vi "NI 5772 (AC) - TIS Mode Enabled (FPGA).vi"() -> ()   [LabVIEW 2018]
doc: "Example Description:\nThis example demonstrates how to enable Time Interleaved Sampling with the NI 5772 adapter module to achieve a sampling rate of 1.6GS/s. This example continuously acquires records of analog input data from the NI 5772 adapter module. It allows you to select an AI channel, trigger type, and record size. This VI must be compiled before it is run. \n\nRunning the VI:\nThis VI must be run from the NI 5772 - Getting Started (Host).vi. Refer to the host VI documentation for steps regarding running and configuring the FPGA VI. \n\nExecution Steps:\nRefer to the Block Diagram of this VI for execution comments."
uses:
  Controls/AI Trigger Type.ctl
  Controls/Aquire State.ctl
  <vilib>/Platform/TimedLoop/XDataNode/timing_clust.ctl
  <vilib>/Platform/TimedLoop/XDataNode/nitl_modes.ctl
  <vilib>/Platform/TimedLoop/XDataNode/wakeup.ctl
  E:/Norway Project/All Hardware/New Microscope/LabVIEW/HardwareRevamp/AcustoXv2/Controls/DigitizerState.ctl
  <instrlib>/_niInstr/Data Trigger/v1/Shared/Public/Edge Configuration Bool.ctl
  <instrlib>/_niInstr/Data Trigger/v1/Shared/Public/Edge Configuration Trigger Slope.ctl
  <vilib>/rvi/Emulation/niFpgaGetClockAttributes.vi
  <vilib>/rvi/Emulation/niFpgaSctlEmulationGetInTimedLoop.vi
  <vilib>/rvi/Emulation/niFpgaEmulationReportErrorSimple.vi
  <vilib>/rvi/eio/common/nirviEmuTemplateMethod_errors.vi
  <vilib>/rvi/Emulation/niFpgaCriticalErrorInLSC.vi
  <vilib>/rvi/Emulation/niFpgaProcessEmulError.vi
  <instrlib>/_niInstr/Data Trigger/v1/FPGA/Private/Trigger/Edge Boolx1spc.vi
  <vilib>/rvi/Emulation/niFpgaEmulationIsFPGAContextNoSignature.vi
  <vilib>/rvi/errors/niFpgaSetErrorForExecOnDevCompSimple.vi
  <vilib>/rvi/eio/common/nirviEmuReportErrorAndStop.vi
  <vilib>/rvi/DataTransferAndStorage/Container/Common/niFpgaContainerGetUniqueNameForEmu.vi
  <vilib>/rvi/FIFO/Fifo_Resource/nirvififoEmulationSetSize.vi
  <vilib>/rvi/FIFO/Fifo_Resource/nirviFifoEmulationQueueMgr.vi
  <instcachedir>/0/nirviFifoEmulationQueueMgr_E5CAEC123FF24DC58D834DCA3CDAA9B5.lvgen/nirviFifoEmulationQueueMgr_E5CAEC123FF24DC58D834DCA3CDAA9B5_003.vi
  <vilib>/rvi/FIFO/Fifo_Resource/nirvififoEmulationDetermineInputValidOut.vi
  <vilib>/rvi/FIFO/Fifo_Resource/nirvififoEmulationCreateLock.vi
  <vilib>/rvi/FIFO/Fifo_Resource/nirvififoEmulationObtainLock.vi
  <vilib>/rvi/FIFO/Fifo_Resource/nirvififoEmulationReleaseLock.vi
  <vilib>/rvi/occurrence/nirviWaitOnOccurrenceBase.vi
  <vilib>/rvi/errors/nirviReportUnexpectedCaseInternalError.vi
  <vilib>/rvi/errors/nirviReportUnexpectedCaseInternalError (U32).vi
  <vilib>/Utility/error.llb/Clear Errors.vi
  <vilib>/rvi/interface/RandomDataEmulation/niFpgaRandomDataHandleErrors.vi
  <vilib>/eio/EIONode/EIONode.xnode
  <vilib>/Platform/TimedLoop/XDataNode/XDataNode.xnode
  <vilib>/rvi/DataTransferAndStorage/Container/XNode/niFpgaContainer.xnode
  <vilib>/rvi/FIFO/Fifo_Resource/nirvififoEmulationWrite.vi
  <vilib>/rvi/FIFO/Fifo_Resource/nirvififoEmulationRead.vi
  <vilib>/rvi/interface/RandomDataEmulation/nirviRandomDataFpgaReadWriteTemplate.vi
  <vilib>/Platform/TimedLoop/XDataNode/XDNodeRunTimeDep.lvlib
  <instrlib>/_niInstr/Data Trigger/v1/FPGA/niInstr Data Trigger v1 FPGA.lvlib
  <instrlib>/_niInstr/Data Trigger/v1/Shared/niInstr Data Trigger v1 Shared.lvlib
panel:
  in  "vi/nGenTrig":bool
  out "Pixel and Wave":T1
  out "Completed?":bool
  in  "Scan Mode":enum16{"Raster Scan", "Serpentine Scan"}(ring)
  in  "Line Count":u16
  in  "Pixel Count":u16
  in  "TrigIn Simulate":bool
  in  "Filteration":bool
  out "DMA FIFO Overflow?":bool caption="FIFO Overflow?"
  in  "AvgCount":u16=1
  in  "Delay after Trig [us]":sgl
  out "Delay after Trig [cycles]":u16
  out "TS FIFO In Overflow?":bool caption="FIFO Overflow?"
  in  "Samples Per Trigger":u16=512 min=1 step=1
  in  "Arm Trigger":bool
  in  "User Command Commit":bool
  in  "User Command":u8
  out "User Command Idle":bool
  out "User Command Status":u8
  in  "User Data 0":u16
  in  "User Data 1":u8
  out "PLL Locked":bool
  out "User Error":bool
  out "Configured?":bool
  in  "Trigger Level":i16
  in  "Trigger Type":T2
  # "Resource Configuration"
  # "Analog Input"
  # "Clock Configuration"
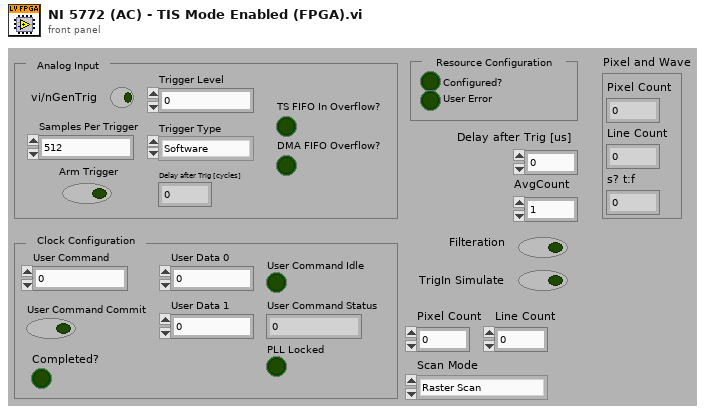
[diagram p1: front panel]
types:
  T1 = cluster{"Pixel Count":i32, "Line Count":u16, "s? t:f":u64}
  T2 = typedef "AI Trigger Type.ctl" = enum8{"Software", "Data Edge"}
  T3 = typedef "DigitizerState.ctl" = enum16{"GetData", "Filter", "AverageCountCheck", "SendtoHost", "CompleteScan"}
  T4 = typedef "Aquire State.ctl" = enum8{"Idle", "Wait for Trigger", "Hold Aquire", "Acquire"}
  T5 = typedef "XDNodeRunTimeDep.lvlib/timing_clust.ctl" = cluster{"Expected End [f-1]":u64, "Actual End [f-1]":u64, "Finished Late? [f-1]":bool, "Expected End [i-1]":u64, "Actual End [i-1]":u64, "Finished Late? [i-1]":bool, "Expected Start [i]":u64, "Actual Start [i]":u64, "Expected Start [f]":u64, "Actual Start [f]":u64, "Source Name":string, "Structure Name":string, "Period":i64, "Deadline":i64, "Offset":i64, "Start":i64, "Priority":i32, "Timeout":i32, "Mode":T6, "Wakeup Reason":T7, "Error":errorcluster, "Source Type":string, "Secondary Source Type":string, "Global End Time":u64, "Global Start Time":u64, "Frame Duration":u64, "Iteration Duration":u64, "Assigned CPU":i32, "I/O Scan Engine Mode":u32}
  T6 = typedef "XDNodeRunTimeDep.lvlib/nitl_modes.ctl" = enum32{"No Change", "Process missed periods, maintain original phase", "Discard missed periods, maintain original phase", "Process missed periods, ignore original phase", "Discard missed periods, ignore original phase"}
  T7 = typedef "XDNodeRunTimeDep.lvlib/wakeup.ctl" = enum32{"Normal", "Aborted", "Asynchronous wakeup", "Timing source error", "Timed loop error", "Timeout"}
  T8 = typedef "niInstr Data Trigger v1 Shared.lvlib/Edge Configuration Bool.ctl" = cluster{"trigger slope":T9}
  T9 = typedef "niInstr Data Trigger v1 Shared.lvlib/Edge Configuration Trigger Slope.ctl" = enum8{"Positive", "Negative"}
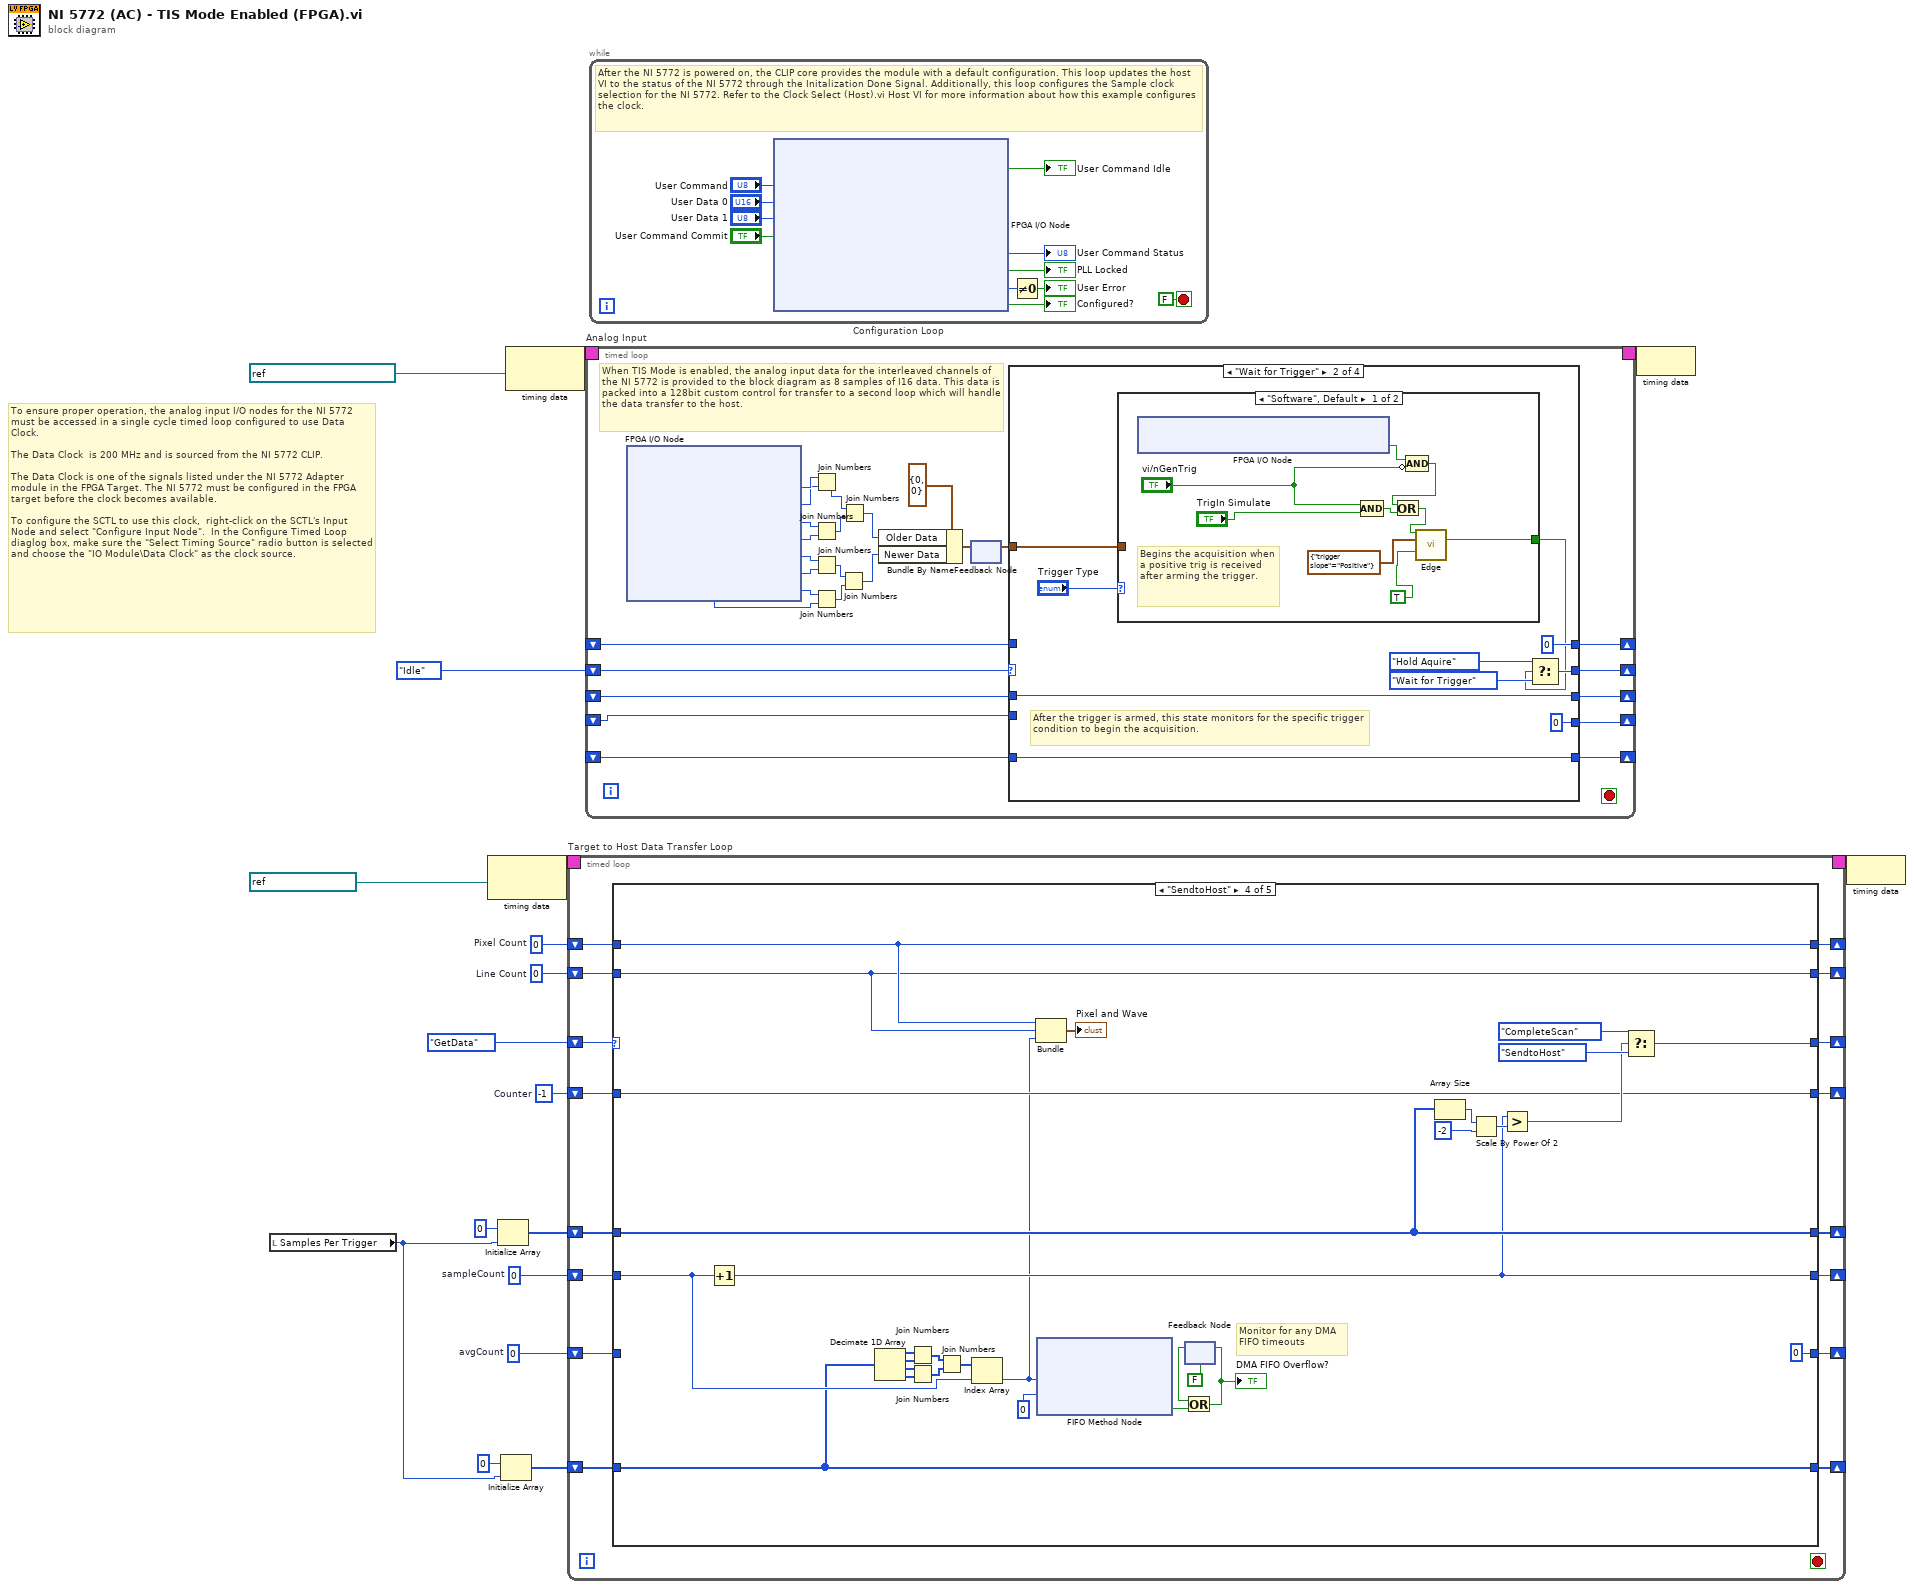
[diagram p0: block diagram]
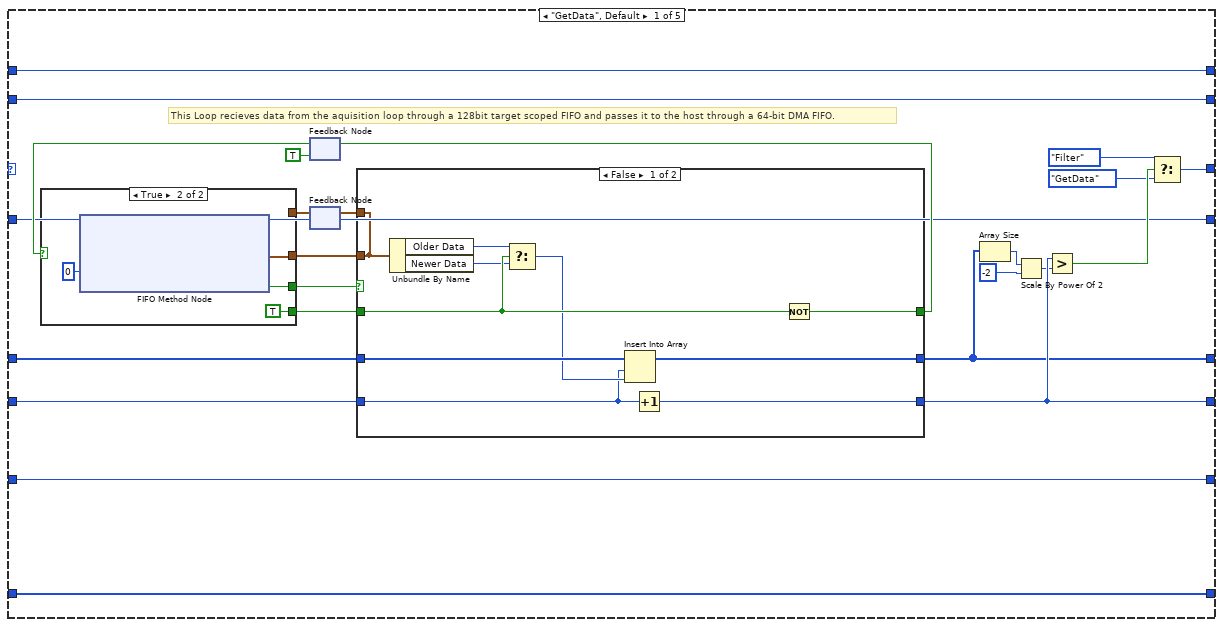
[diagram p2: hidden frame]
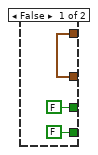
[diagram p3: hidden frame]
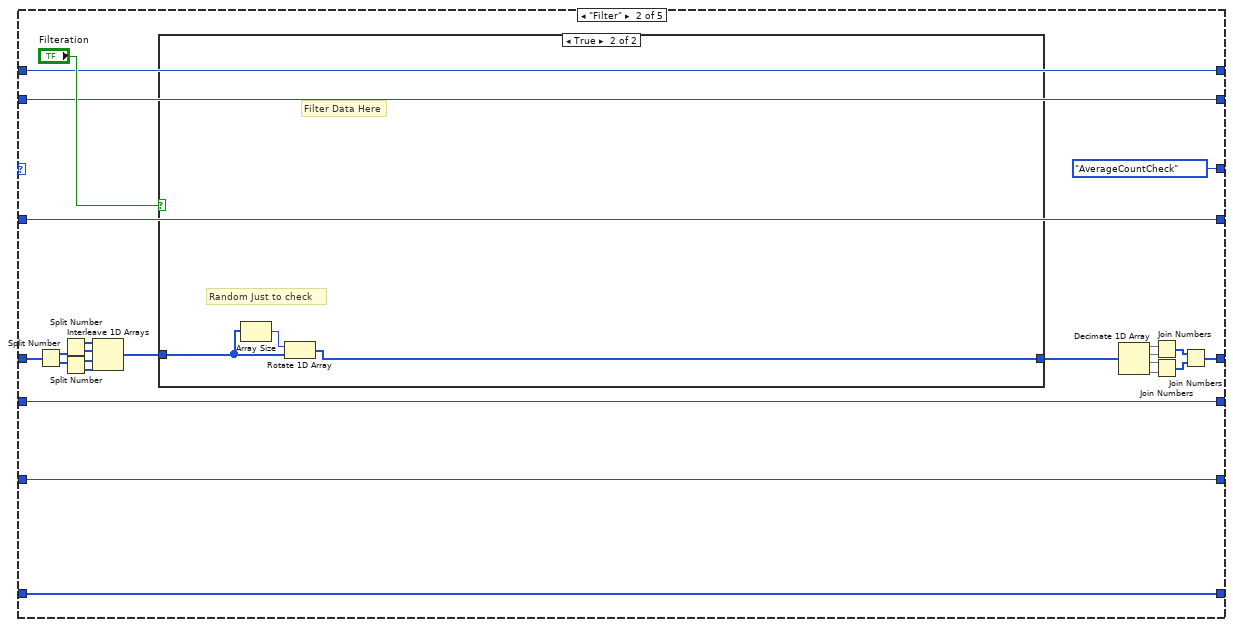
[diagram p5: hidden frame]
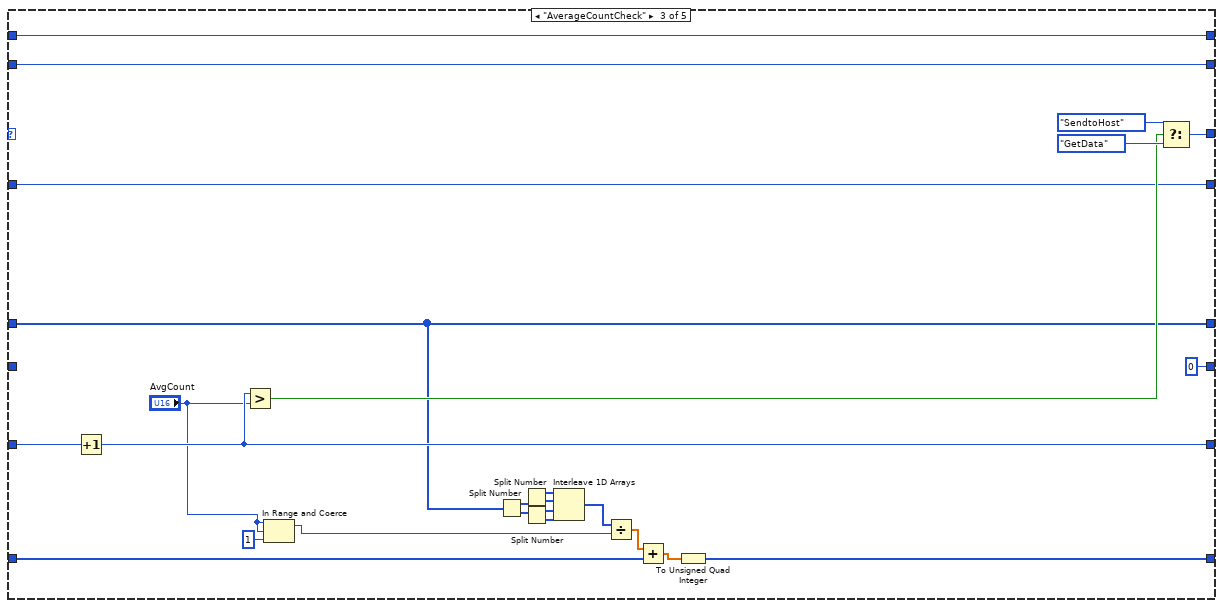
[diagram p7: hidden frame]
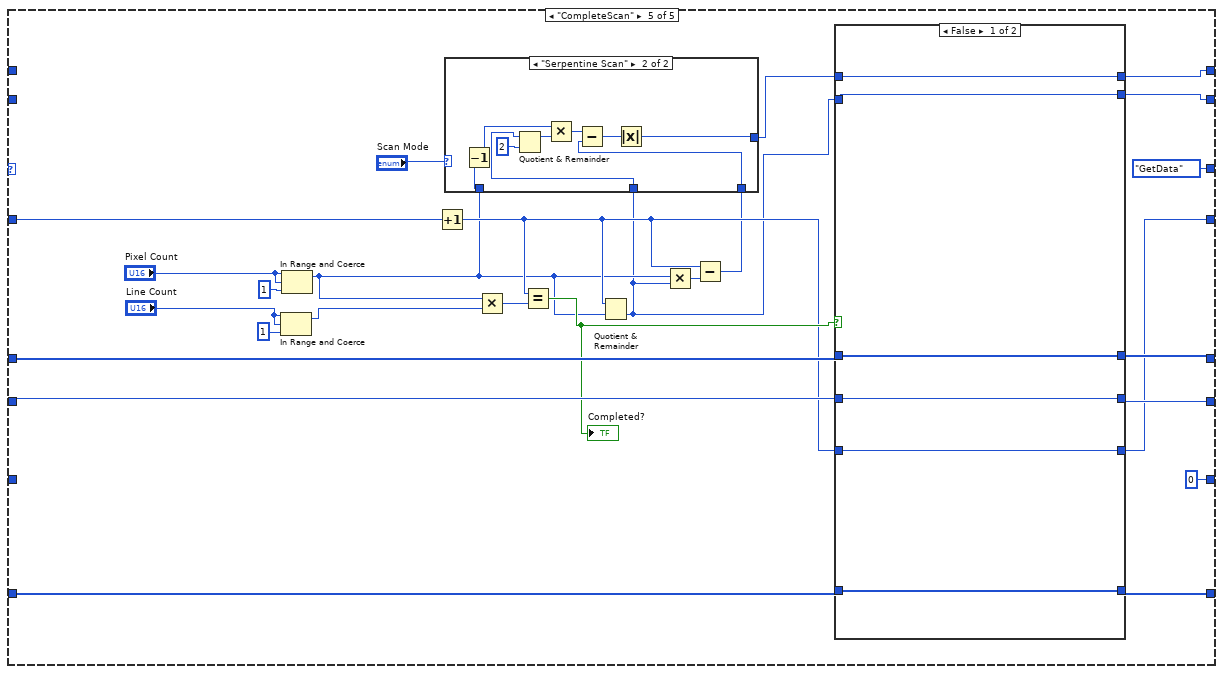
[diagram p8: hidden frame]
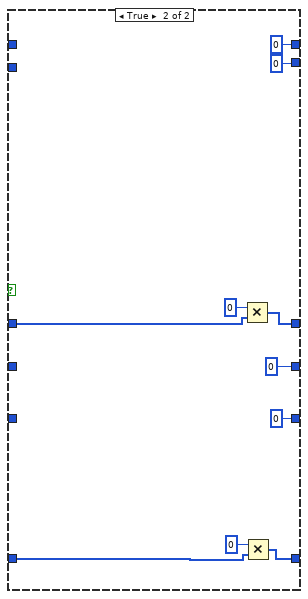
[diagram p10: hidden frame]
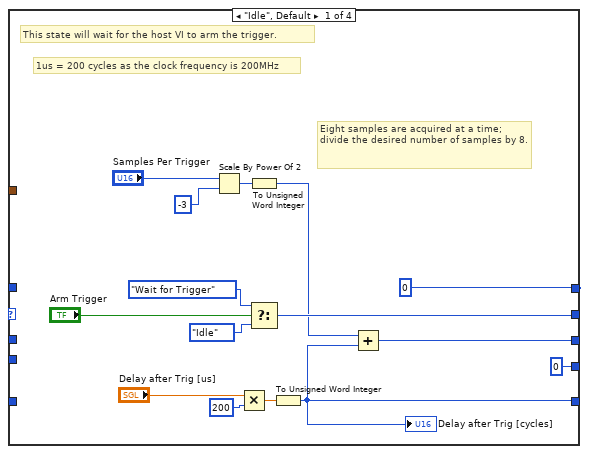
[diagram p11: hidden frame]
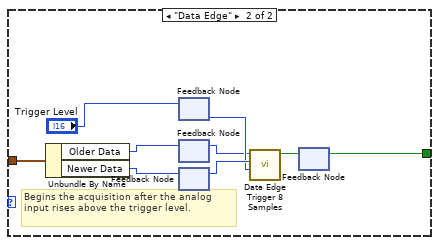
[diagram p12: hidden frame]
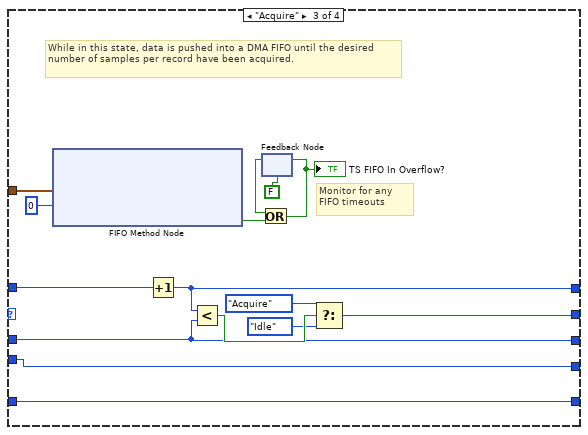
[diagram p13: hidden frame]
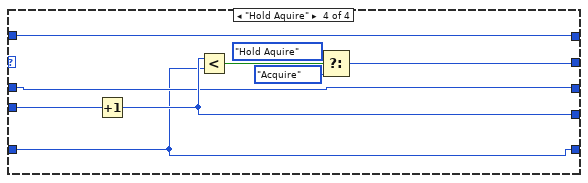
[diagram p14: hidden frame]
diagram:
  w1 = i16 -1  # Counter
  w2 = u16 0  # Line Count
  w3 = u16 0  # Pixel Count
  w7 = u16 0  # avgCount
  w8 = u16 0  # sampleCount
  # "To ensure proper operation, the analog input I/O nodes for the NI 5772 must be accessed in a single cycle timed loop configured to use Data Clock. \n\nThe Data Clock  is 200 MHz and is sourced from the NI 5772 CLIP.\n\nThe Data Clock is one of the signals listed under the NI 5772 Adapter module in the FPGA Target. The NI 5772 must be configured in the FPGA target before the clock becomes available. \n\nTo configure the SCTL to use this clock,  right-click on the SCTL's Input Node and select \"Configure Input Node\".  In the Configure Timed Loop diaglog box, make sure the \"Select Timing Source\" radio button is selected and choose the \"IO Module\\Data Clock\" as the clock source."
  n1 = local read "Samples Per Trigger"() -> (w4:u16)
  n2 = node-c288(refnum<k21> "100 MHz Clock" ("Source Name")) -> (w16:T5)
  n3 = Initialize Array(u64 0 ("s? t:f"), w4) -> (w9:u64[])
  n4 = Initialize Array(u64 0 ("s? t:f"), w4) -> (w5:u64[])
  n5 = node-c288(refnum<k21> "IO Module\\Data Clock" ("Source Name")) -> (w18:T5)
  n6 = timed-loop "Target to Host Data Transfer Loop" {
    timing: w16 -> [_]
    timing-out: [_] -> w15
    shift-right: [w29] -> _
    shift-left: DigitizerState."GetData" -> [w34]
    shift-right: [w32] -> _
    shift-left: w9 -> [w33]
    shift-right: [w30] -> _
    shift-left: w8 -> [w31]
    shift-right: [w25] -> _
    shift-left: w7 -> [w28]
    shift-right: [w26] -> _
    shift-left: w5 -> [w27]
    shift-right: [w22] -> _
    shift-left: w3 -> [w24]
    shift-right: [w21] -> _
    shift-left: w2 -> [w23]
    shift-right: [w19] -> _
    shift-left: w1 -> [w20]
    stop <- _ stop-if-true
    n7 = case shown="\"SendtoHost\"" w34 {
      tunnel: w33 -> [w58 w93 w117 w140 w186]
      tunnel: [w41 w87 w117 w140 w185] -> w32
      tunnel: w31 -> [w57 w103 _ w149 w182]
      tunnel: [w48 w103 u16 0 ("sampleCount") w139 w184] -> w30
      tunnel: [w44 DigitizerState."AverageCountCheck" w128 w146 DigitizerState."GetData"] -> w29
      tunnel: w28 -> [w42 w102 w132 _ _]
      tunnel: w27 -> [w43 w101 w125 w138 w181]
      tunnel: [w43 w101 w124 w138 w183] -> w26
      tunnel: [w42 w102 w131 u16 0 ("sampleCount") u16 0 ("sampleCount")] -> w25
      tunnel: w24 -> [w37 w82 w110 w135 _]
      tunnel: w23 -> [w36 w81 w109 w134 _]
      tunnel: [w37 w82 w110 w135 w166] -> w22
      tunnel: [w36 w81 w109 w134 w165] -> w21
      tunnel: w20 -> [w35 w80 w108 w137 w177]
      tunnel: [w35 w80 w108 w137 w173] -> w19
      frame "GetData", Default {
        # "This Loop recieves data from the aquisition loop through a 128bit target scoped FIFO and passes it to the host through a 64-bit DMA FIFO."
        n8 = feedback #1(TRUE ("Timed Out?")) -> (w54:bool)
        n9 = feedback #2() -> (w53:cluster{"Older Data":u64, "Newer Data":u64})  [unwired: 1 in]
        n10 = case shown="True" w54 {
          tunnel: [w59 w62] -> w51
          tunnel: [FALSE ("Timed Out?") w63] -> w50
          tunnel: [FALSE ("Timed Out?") TRUE ("Timed Out?")] -> w49
          tunnel: w53 -> [w59 _]
          frame False {
          }
          frame True {
            n11 = xnode ("FIFO Method Node")("Timeout"=0) -> ("Element"=w62:cluster{"Older Data":u64, "Newer Data":u64}, "Timed Out?"=w63:bool)  [unwired: 1 in, 1 out]
          }
        }
        n12 = case shown="False" w50 {
          tunnel: [w73 w79] -> w55
          tunnel: w49 -> [w74 w79]
          tunnel: w51 -> [w72 w78]
          tunnel: [w72 w78] -> w52
          tunnel: w57 -> [w66 w77]
          tunnel: [w70 w77] -> w48
          tunnel: w58 -> [w69 w76]
          tunnel: [w68 w76] -> w41
          frame False {
            n13 = Unbundle By Name(w72) -> ("Older Data"=w75:u64, "Newer Data"=w71:u64)
            n14 = Select(t=w75, s=w74, f=w71) -> (s? t:f=w67:u64)
            n15 = Insert Into Array(array=w69, index=w66, new element=w67) -> (w68:u64[])
            n16 = Increment(x=w66) -> (x+1=w70:u16)
            n17 = Not(x=w74) -> (.not. x?=w73:bool)
          }
          frame True {
          }
        }
        n18 = feedback-in #1(w55) -> ()
        n19 = feedback-in #2(w52) -> ()
        n20 = Array Size(array=w41) -> (size(s)=w39:i32)
        n21 = Scale By Power Of 2(n=w39, x=i8 -2 ("y")) -> (x*2^n=w38:i8)
        n22 = Greater?(x=w48, y=w38) -> (0:w47:bool)
        n23 = Select(t=DigitizerState."Filter", s=w47, f=DigitizerState."GetData") -> (s? t:f=w44:T3)
      }
      frame "Filter" {
        n24 = Split Number(x=w93) -> (hi(x)=w95:u32[], lo(x)=w96:u32[])
        n25 = Split Number(x=w95) -> (hi(x)=w94:u16[], lo(x)=w99:u16[])
        n26 = Split Number(x=w96) -> (hi(x)=w98:u16[], lo(x)=w97:u16[])
        n27 = Interleave 1D Arrays(w94, w99, w98, w97) -> (w85:u16[])
        n28 = case shown="True" "Filteration" {
          tunnel: w85 -> [w104 w105]
          tunnel: [w104 w107] -> w84
          frame False {
          }
          frame True {
            # "Random Just to check"
            # "Filter Data Here"
            n29 = Array Size(array=w105) -> (size(s)=w106:i32)
            n30 = Rotate 1D Array(1:w105, 2:w106) -> (0:w107:u16[])
          }
        }
        n31 = Decimate 1D Array(w84) -> (w92:u16[], w91:u16[], w90:u16[], w83:u16[])
        n32 = Join Numbers(hi=w92, lo=w91) -> ((hi.lo)=w89:u32[])
        n33 = Join Numbers(hi=w90, lo=w83) -> ((hi.lo)=w88:u32[])
        n34 = Join Numbers(hi=w89, lo=w88) -> ((hi.lo)=w87:u64[])
      }
      frame "AverageCountCheck" {
        n35 = Increment(x=w132) -> (x+1=w131:u16)
        n36 = Greater?(x=w131, y="AvgCount") -> (0:w127:bool)
        n37 = In Range and Coerce(upper limit="AvgCount", x="AvgCount", lower limit=u16 1) -> (coerced(x)=w111:u16)  [unwired: 1 out]
        n38 = Split Number(x=w117) -> (hi(x)=w118:u32[], lo(x)=w119:u32[])
        n39 = Split Number(x=w118) -> (hi(x)=w116:u16[], lo(x)=w122:u16[])
        n40 = Split Number(x=w119) -> (hi(x)=w121:u16[], lo(x)=w120:u16[])
        n41 = Interleave 1D Arrays(w116, w122, w121, w120) -> (w112:u16[])
        n42 = Divide(x=w112, y=w111) -> (x/y=w113:sgl[])
        n43 = Add(x=w113, y=w125) -> (x+y=w123:sgl[])
        n44 = To Unsigned Quad Integer(1:w123) -> (0:w124:u64[])
        n45 = Select(t=DigitizerState."SendtoHost", s=w127, f=DigitizerState."GetData") -> (s? t:f=w128:T3)
      }
      frame "SendtoHost" {
        # "Monitor for any DMA FIFO timeouts"
        n46 = Increment(x=w149) -> (x+1=w139:u16)
        n47 = Decimate 1D Array(w138) -> (w155:u64[], w154:u64[], w153:u64[], w152:u64[])
        n48 = Join Numbers(hi=w155, lo=w154) -> ((hi.lo)=w151:u64[])
        n49 = Join Numbers(hi=w153, lo=w152) -> ((hi.lo)=w150:u64[])
        n50 = Join Numbers(hi=w151, lo=w150) -> ((hi.lo)=w144:u64[])
        n51 = Index Array(array=w144, index=w149) -> (element=w136:u64)
        n52 = Bundle("Pixel Count"=w135, "Line Count"=w134, "s? t:f"=w136) -> (→"Pixel and Wave":T1)  [unwired: 1 in]
        n53 = xnode ("FIFO Method Node")("Element"=w136, "Timeout"=0) -> ("Timed Out?"=w157:bool)  [unwired: 1 in, 1 out]
        n54 = feedback #3(FALSE) -> (w160:bool)
        n55 = Or(x=w160, y=w157) -> (x .or. y?=w158:bool)
        "DMA FIFO Overflow?" <- w158
        n56 = feedback-in #3(w158) -> ()
        n57 = Array Size(array=w140) -> (size(s)=w142:i32)
        n58 = Scale By Power Of 2(n=w142, x=i8 -2 ("y")) -> (x*2^n=w141:i8)
        n59 = Greater?(x=w139, y=w141) -> (0:w145:bool)
        n60 = Select(t=DigitizerState."CompleteScan", s=w145, f=DigitizerState."SendtoHost") -> (s? t:f=w146:T3)
      }
      frame "CompleteScan" {
        n61 = In Range and Coerce(upper limit="Line Count", x="Line Count", lower limit=u16 1) -> (coerced(x)=w167:u16)  [unwired: 1 out]
        n62 = In Range and Coerce(upper limit="Pixel Count", x="Pixel Count", lower limit=u16 1) -> (coerced(x)=w170:u16)  [unwired: 1 out]
        n63 = Increment(x=w177) -> (x+1=w174:i16)
        n64 = Multiply(x=w170, y=w167) -> (x*y=w179:u16)
        n65 = Equal?(x=w174, y=w179) -> (x = y?=w175:bool)
        "Completed?" <- w175
        n66 = Quotient & Remainder(x=w174, y=w170) -> (floor(x/y)=w163:u16)  [unwired: 1 out]
        n67 = Multiply(x=w170, y=w163) -> (x*y=w180:u16)
        n68 = Subtract(x=w174, y=w180) -> (x-y=w162:u16)
        n69 = case shown="\"Serpentine Scan\"" "Scan Mode" {
          tunnel: w162 -> [w188 w192]
          tunnel: [w188 w190] -> w164
          tunnel: w163 -> [_ w197]
          tunnel: w170 -> [_ w195]
          frame "Raster Scan", Default {
          }
          frame "Serpentine Scan" {
            n70 = Decrement(x=w195) -> (x-1=w189:u16)
            n71 = Quotient & Remainder(x=w197, y=2) -> (x-y*floor(x/y)=w194:i32)  [unwired: 1 out]
            n72 = Multiply(x=w189, y=w194) -> (x*y=w193:i32)
            n73 = Subtract(x=w193, y=w192) -> (x-y=w191:i32)
            n74 = Absolute Value(x=w191) -> (abs(x)=w190:i32)
          }
        }
        n75 = case shown="False" w175 {
          tunnel: [w203 u16 0] -> w184
          tunnel: w182 -> [w203 _]
          tunnel: w181 -> [w202 w207]
          tunnel: w186 -> [w201 w208]
          tunnel: [w201 w211] -> w185
          tunnel: [w202 w209] -> w183
          tunnel: w174 -> [w200 _]
          tunnel: [w200 i16 0] -> w173
          tunnel: w164 -> [w199 _]
          tunnel: [w199 0] -> w166
          tunnel: w163 -> [w198 _]
          tunnel: [w198 u16 0] -> w165
          frame False {
          }
          frame True {
            n76 = Multiply(x=u64 0 ("s? t:f"), y=w208) -> (x*y=w211:u64[])
            n77 = Multiply(x=u64 0 ("s? t:f"), y=w207) -> (x*y=w209:u64[])
          }
        }
      }
    }
  }
  n78 = timed-loop "Analog Input" {
    timing: w18 -> [_]
    timing-out: [_] -> w17
    shift-right: [w241] -> _
    shift-left: Aquire_State."Idle" ("Acquire State") -> [w231]
    shift-right: [w242] -> _
    shift-left: _ -> [w232]
    shift-right: [w240] -> _
    shift-left: _ -> [w230]
    shift-right: [w219] -> _
    shift-left: _ -> [w218]
    shift-right: [w216] -> _
    shift-left: _ -> [w217]
    stop <- _ stop-if-true
    # "When TIS Mode is enabled, the analog input data for the interleaved channels of the NI 5772 is provided to the block diagram as 8 samples of I16 data. This data is packed into a 128bit custom control for transfer to a second loop which will handle the data transfer to the host."
    n79 = xnode "FPGA I/O Node"() -> ("IO Module\\AI 1 Data N-3"=w223:i16, "IO Module\\AI 0 Data N-3"=w222:i16, "IO Module\\AI 1 Data N-2"=w221:i16, "IO Module\\AI 0 Data N-2"=w220:i16, "IO Module\\AI 1 Data N-1"=w224:i16, "IO Module\\AI 0 Data N-1"=w225:i16, "IO Module\\AI 1 Data N"=w226:i16, "IO Module\\AI 0 Data N"=w227:i16)  [unwired: 8 in, 8 out]
    n80 = Join Numbers(hi=w223, lo=w222) -> ((hi.lo)=w235:u32)
    n81 = Join Numbers(hi=w221, lo=w220) -> ((hi.lo)=w237:u32)
    n82 = Join Numbers(hi=w224, lo=w225) -> ((hi.lo)=w236:u32)
    n83 = Join Numbers(hi=w226, lo=w227) -> ((hi.lo)=w238:u32)
    n84 = Join Numbers(hi=w236, lo=w238) -> ((hi.lo)=w228:u64)
    n85 = Join Numbers(hi=w235, lo=w237) -> ((hi.lo)=w229:u64)
    n86 = Bundle By Name(cluster=cluster{"Older Data":u64, "Newer Data":u64} {"Older Data"=0, "Newer Data"=0} ("Element"), "Older Data"=w229, "Newer Data"=w228) -> (w233:cluster{"Older Data":u64, "Newer Data":u64})
    n87 = feedback #4() -> (w239:cluster{"Older Data":u64, "Newer Data":u64})  [unwired: 1 in]
    n88 = feedback-in #4(w233) -> ()
    n89 = case shown="\"Wait for Trigger\"" w231 {
      tunnel: [u16 0 u16 0 w300 w303] -> w242
      tunnel: w232 -> [_ _ w299 w303]
      tunnel: [w254 w262 w297 w306] -> w241
      tunnel: [w251 w266 w294 w302] -> w240
      tunnel: w230 -> [_ w266 w294 w302]
      tunnel: w239 -> [_ w265 w293 _]
      tunnel: [u16 0 ("Delay after Trig [cycles]") u16 0 ("Delay after Trig [cycles]") w287 w304] -> w219
      tunnel: w218 -> [_ _ w287 w305]
      tunnel: w217 -> [_ w258 w286 w301]
      tunnel: [w246 w258 w286 w301] -> w216
      frame "Idle", Default {
        # "Eight samples are acquired at a time; divide the desired number of samples by 8."
        # "1us = 200 cycles as the clock frequency is 200MHz"
        # "This state will wait for the host VI to arm the trigger."
        n90 = Scale By Power Of 2(n="Samples Per Trigger", x=i8 -3) -> (x*2^n=w245:i8)
        n91 = Multiply(x="Delay after Trig [us]", y=u16 200 ("Delay after Trig [cycles]")) -> (x*y=w248:sgl)
        n92 = To Unsigned Word Integer(number=w245) -> (unsigned 16bit integer=w244:u16)
        n93 = Select(t=Aquire_State."Wait for Trigger" ("Acquire State"), s="Arm Trigger", f=Aquire_State."Idle" ("Acquire State")) -> (s? t:f=w254:T4)
        n94 = To Unsigned Word Integer(number=w248) -> (unsigned 16bit integer=w246:u16)
        "Delay after Trig [cycles]" <- w246
        n95 = Add(x=w244, y=w246) -> (x+y=w251:u16)
      }
      frame "Wait for Trigger" {
        # "After the trigger is armed, this state monitors for the specific trigger condition to begin the acquisition."
        n96 = case shown="\"Software\", Default" "Trigger Type" {
          tunnel: w265 -> [_ w285]
          tunnel: [w276 w277] -> w260
          frame "Software", Default {
            # "Begins the acquisition when a positive trig is received after arming the trigger."
            n97 = xnode "FPGA I/O Node"() -> ("IO Module\\Asynchronous Trigger Input"=w272:bool)  [unwired: 1 in, 1 out]
            n98 = Compound Arithmetic op=AND("vi/nGenTrig", "TrigIn Simulate") -> (w268:bool)
            n99 = Compound Arithmetic op=AND(w272, invert "vi/nGenTrig") -> (w271:bool)
            n100 = Or(x=w271, y=w268) -> (x .or. y?=w273:bool)
            n101 = call-poly <instrlib>:"Edge.vi"("data in"=w273, "configuration"=T8 {"trigger slope"=enum."Positive"}, "input valid"=TRUE) -> ("trigger"=w276:bool)  [unwired: 7 in, 5 out]
          }
          frame "Data Edge" {
            # "Begins the acquisition after the analog input rises above the trigger level."
            n102 = Unbundle By Name(w285) -> ("Older Data"=w283:u64, "Newer Data"=w281:u64)
            n103 = feedback-in #5("Trigger Level") -> ()
            n104 = feedback #5() -> (w279:i16)  [unwired: 1 in]
            n105 = feedback-in #6(w283) -> ()
            n106 = feedback #6() -> (w278:u64)  [unwired: 1 in]
            n107 = feedback-in #7(w281) -> ()
            n108 = feedback #7() -> (w280:u64)  [unwired: 1 in]
            n109 = call "Data Edge Trigger 8 Samples.vi"("Trigger Level"=w279, "Newer Data In"=w280, "Older Data In"=w278) -> ("Trigger"=w284:bool)  [unwired: 8 in]
            n110 = feedback-in #8(w284) -> ()
            n111 = feedback #8() -> (w277:bool)  [unwired: 1 in]
          }
        }
        n112 = Select(t=Aquire_State."Hold Aquire" ("Acquire State"), s=w260, f=Aquire_State."Wait for Trigger") -> (s? t:f=w262:T4)
      }
      frame "Acquire" {
        # "Monitor for any  FIFO timeouts"
        # "While in this state, data is pushed into a DMA FIFO until the desired number of samples per record have been acquired."
        n113 = xnode ("FIFO Method Node")("Element"=w293, "Timeout"=0) -> ("Timed Out?"=w288:bool)  [unwired: 1 in, 1 out]
        n114 = Increment(x=w299) -> (x+1=w300:u16)
        n115 = Less?(x=w300, y=w294) -> (x < y?=w298:bool)
        n116 = feedback #9(FALSE) -> (w289:bool)
        n117 = Or(x=w289, y=w288) -> (x .or. y?=w290:bool)
        "TS FIFO In Overflow?" <- w290
        n118 = feedback-in #9(w290) -> ()
        n119 = Select(t=Aquire_State."Acquire" ("Acquire State"), s=w298, f=Aquire_State."Idle" ("Acquire State")) -> (s? t:f=w297:T4)
      }
      frame "Hold Aquire" {
        n120 = Increment(x=w305) -> (x+1=w304:u16)
        n121 = Less?(x=w304, y=w301) -> (x < y?=w309:bool)
        n122 = Select(t=Aquire_State."Hold Aquire" ("Acquire State"), s=w309, f=Aquire_State."Acquire" ("Acquire State")) -> (s? t:f=w306:T4)
      }
    }
  }
  n123 = while "Configuration Loop" {
    stop <- FALSE stop-if-true
    # "After the NI 5772 is powered on, the CLIP core provides the module with a default configuration. This loop updates the host VI to the status of the NI 5772 through the Initalization Done Signal. Additionally, this loop configures the Sample clock selection for the NI 5772. Refer to the Clock Select (Host).vi Host VI for more information about how this example configures the clock."
    n124 = xnode "FPGA I/O Node"("IO Module\\User Command"="User Command", "IO Module\\User Data 0"="User Data 0", "IO Module\\User Data 1"="User Data 1", "IO Module\\User Command Commit"="User Command Commit") -> ("IO Module\\User Command Idle"=→"User Command Idle":bool, "IO Module\\User Command Status"=→"User Command Status":u8, "IO Module\\PLL Locked"=→"PLL Locked":bool, "IO Module\\User Error"=w317:u8, "IO Module\\Initialization Done"=→"Configured?":bool)  [unwired: 9 in, 9 out]
    n125 = Not Equal To 0?(x=w317) -> (x != 0?=→"User Error":bool)
  }
  n126 = node-c288(w17) -> ()
  n127 = node-c288(w15) -> ()
